vi "Config main.vi"() -> ()   [LabVIEW 2025]
panel:
  in  "Profile Creation":bool
  in  "BATTERY EMULATOR":bool
  in  "CAN CONF":bool
  in  "Configuration":bool
  in  "Home":bool
  in  "Data Log":bool
  in  "Limit Config":bool
  in  "Calibration1":bool
  in  "IO Config":bool
  # "CONFIGURATION"
  # "SETTINGS"
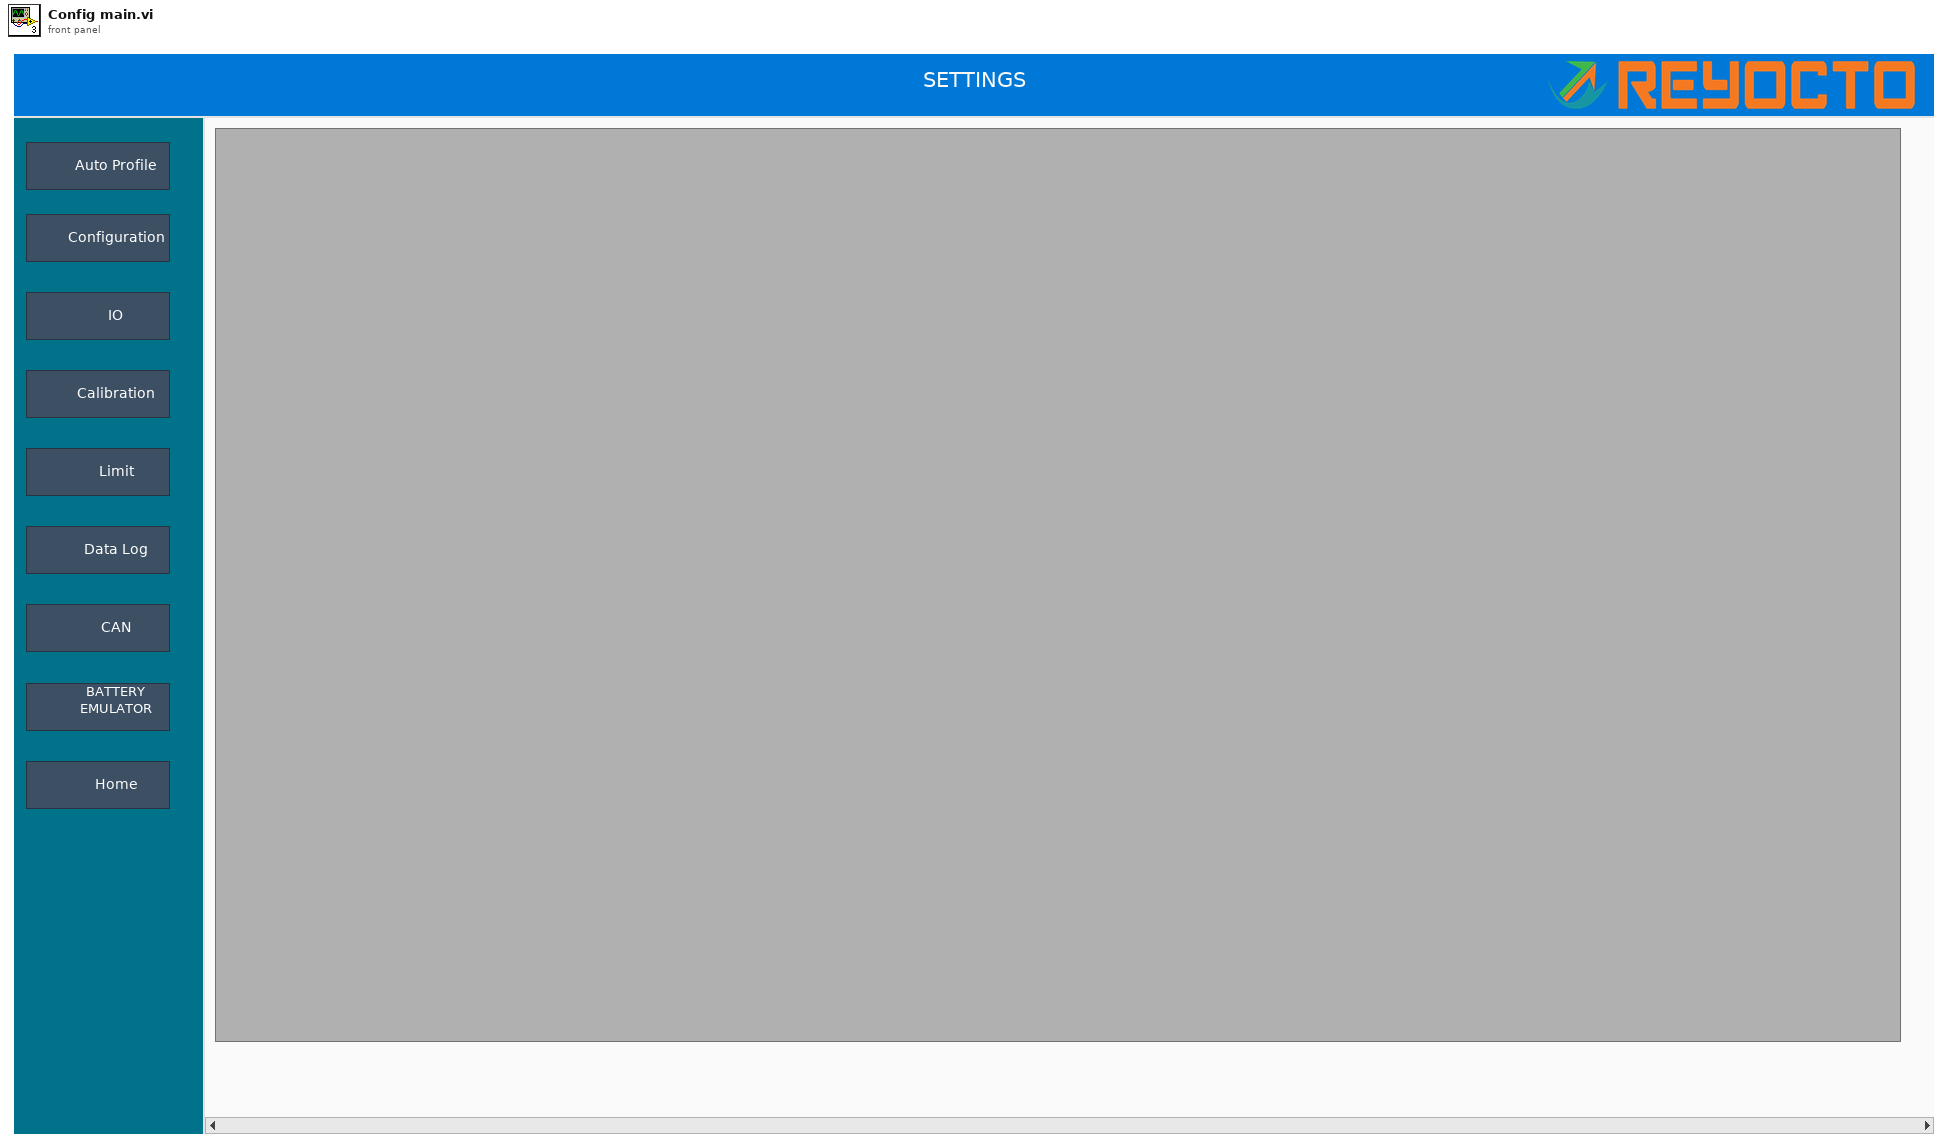
[diagram p1: front panel]
types:
  T1 = enum32{"invalid app kind", "Development System", "Run Time System", "Student Edition", "Embedded LabVIEW", "Evaluation", "Custom"}
  T2 = enum32{"Invalid", "Standard", "Closed", "Hidden", "Minimized", "Maximized"}
  T3 = cluster{"Core":cluster{"Current VI Reference":refnum<vi>, "Close Panel on Exit?":bool}, "Sub Panel":refnum<vi>, "Slected VI":string, "Vi Path":path}
  T4 = cluster{"Current VI Reference":refnum<vi>, "Close Panel on Exit?":bool}
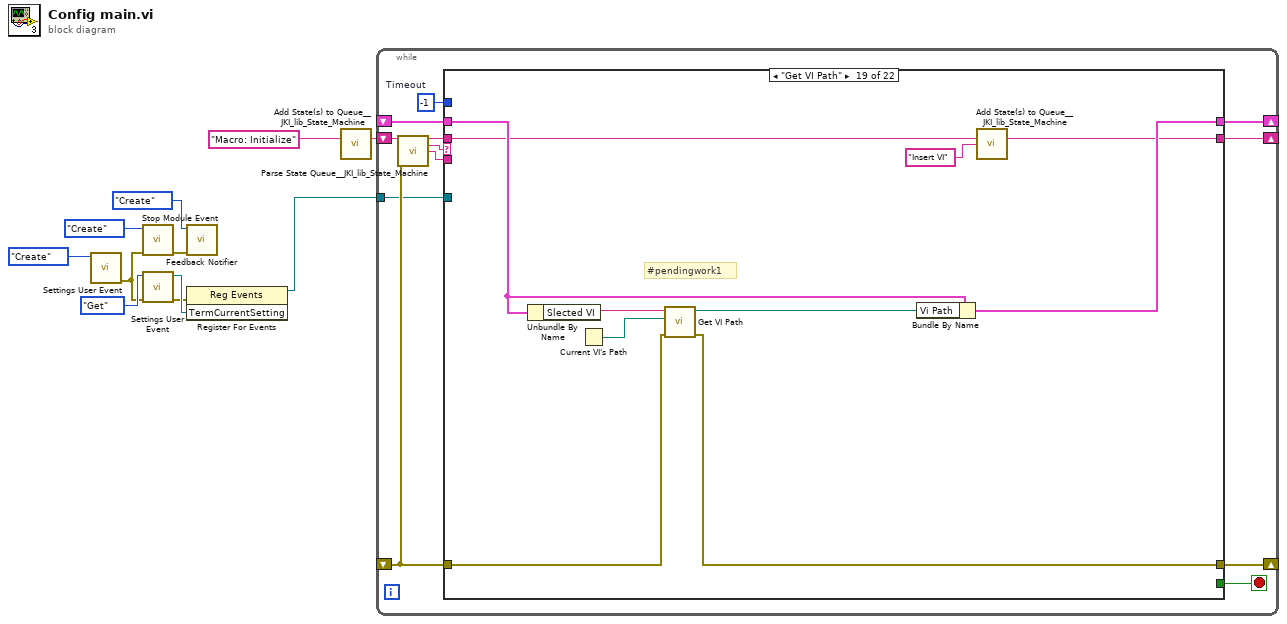
[diagram p0: block diagram]
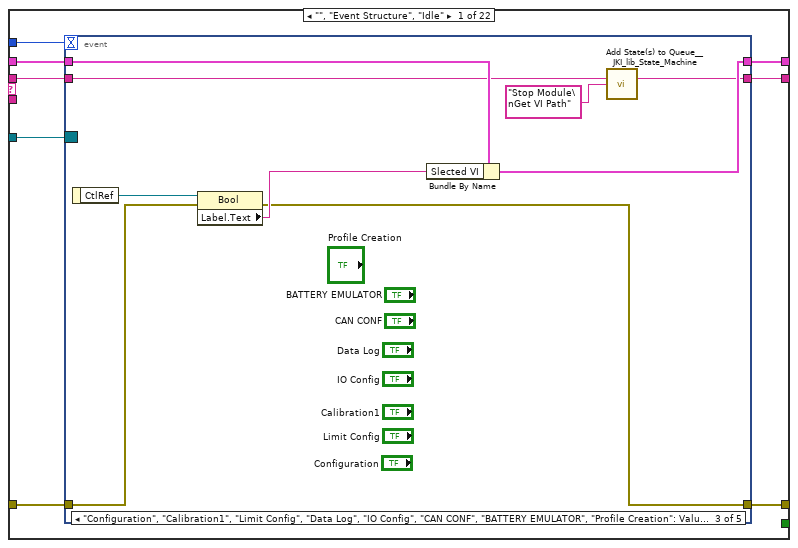
[diagram p2: hidden frame]
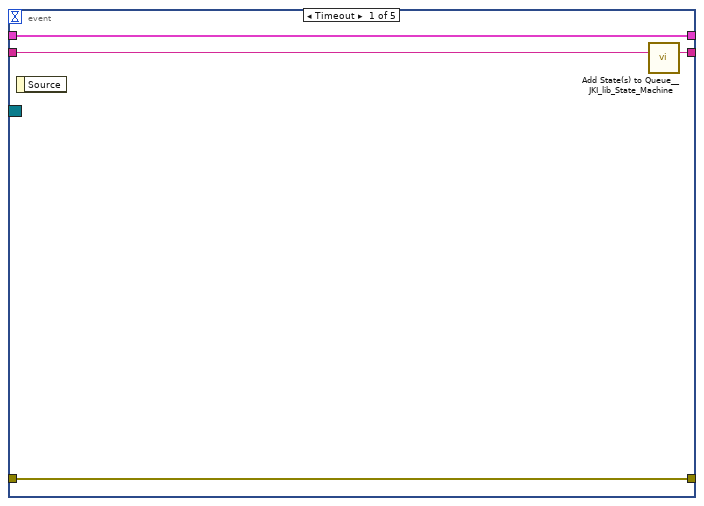
[diagram p3: hidden frame]
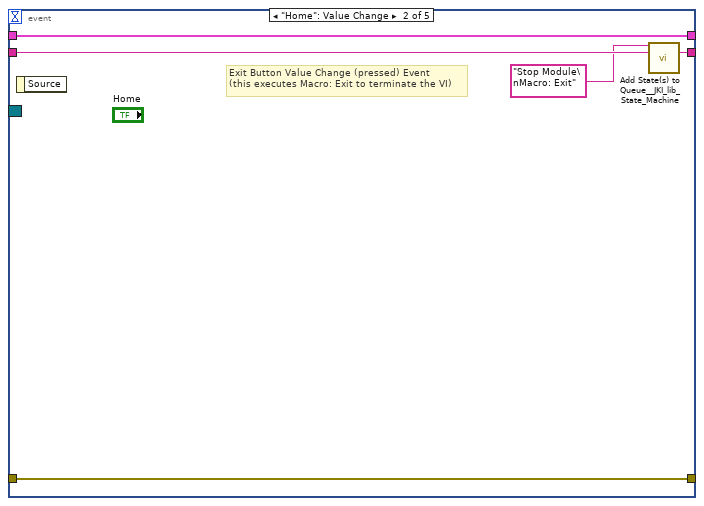
[diagram p4: hidden frame]
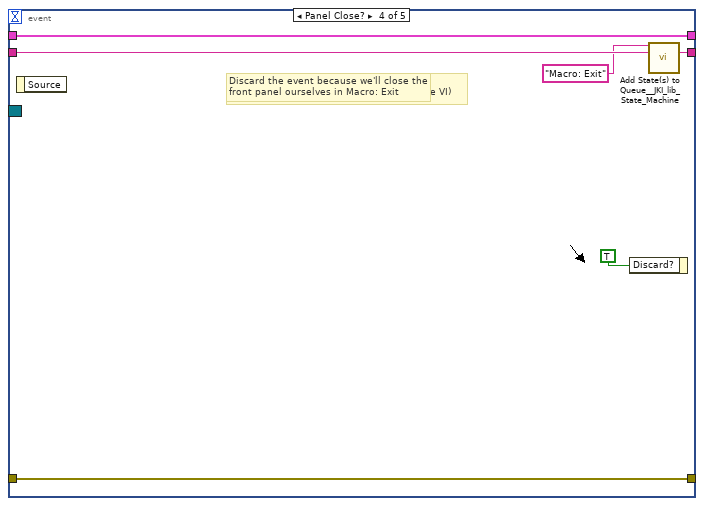
[diagram p5: hidden frame]
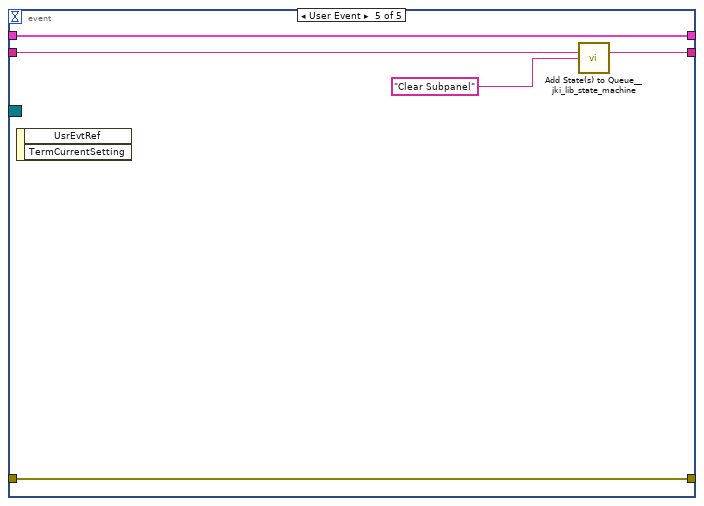
[diagram p6: hidden frame]
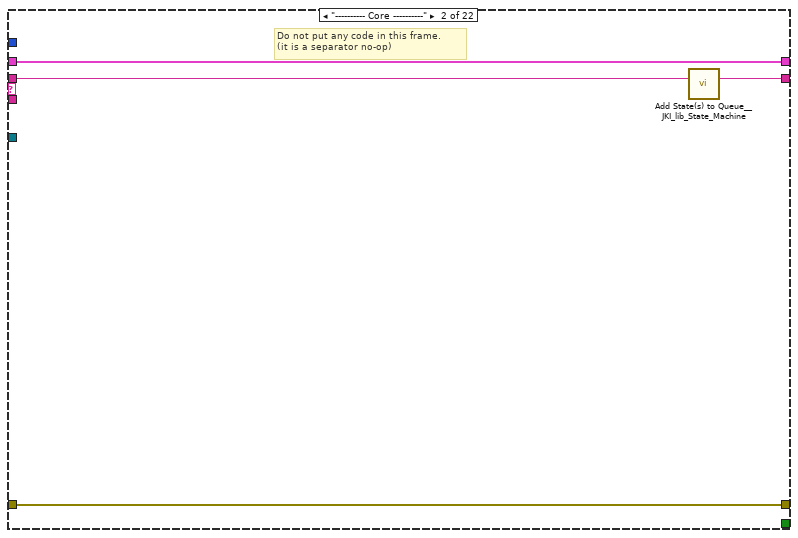
[diagram p7: hidden frame]
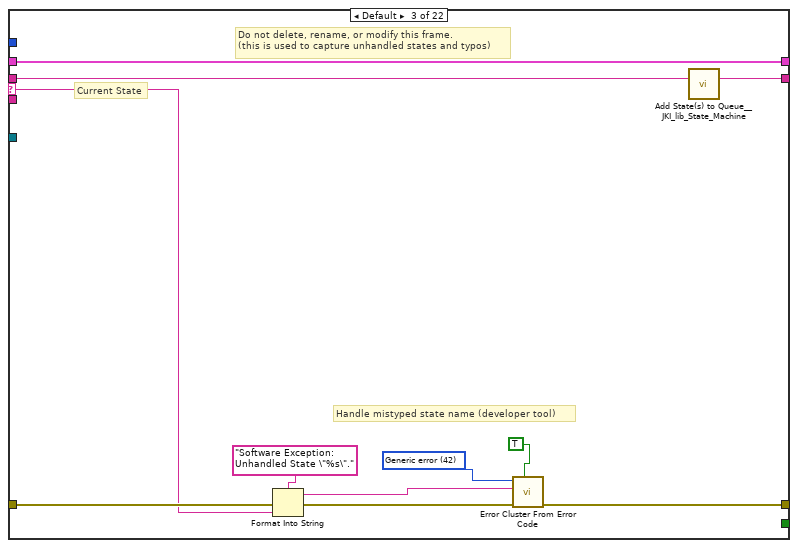
[diagram p8: hidden frame]
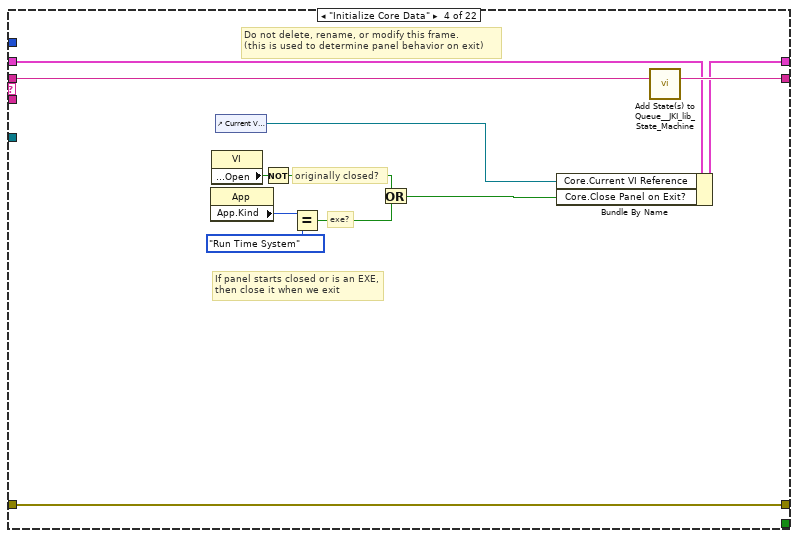
[diagram p9: hidden frame]
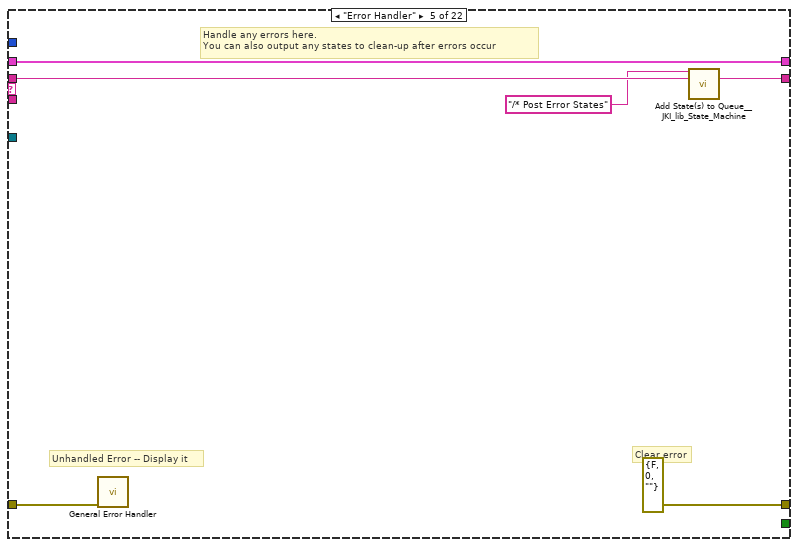
[diagram p10: hidden frame]
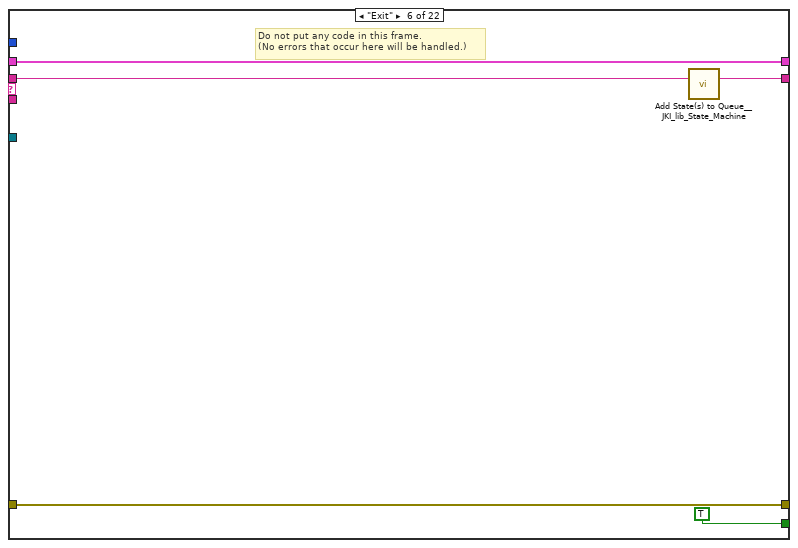
[diagram p11: hidden frame]
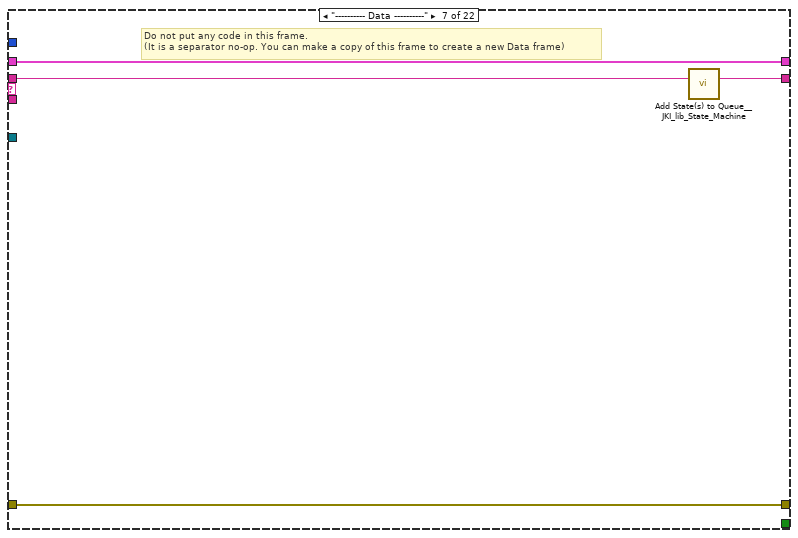
[diagram p12: hidden frame]
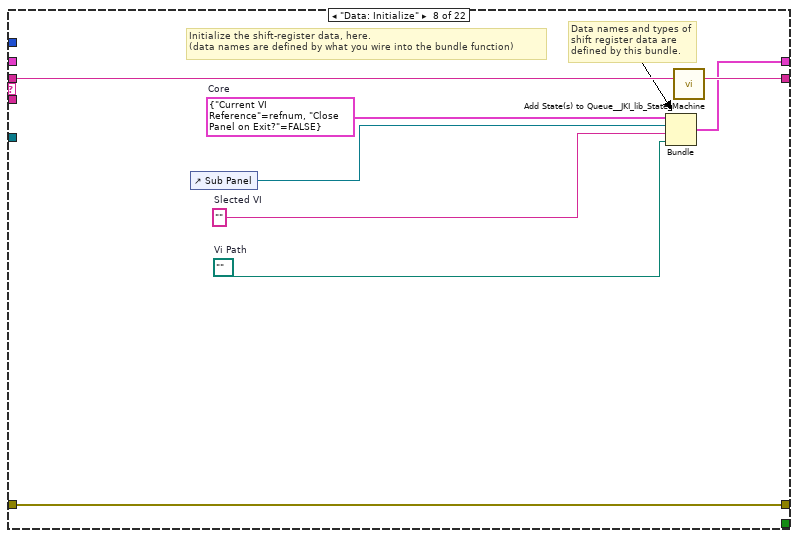
[diagram p13: hidden frame]
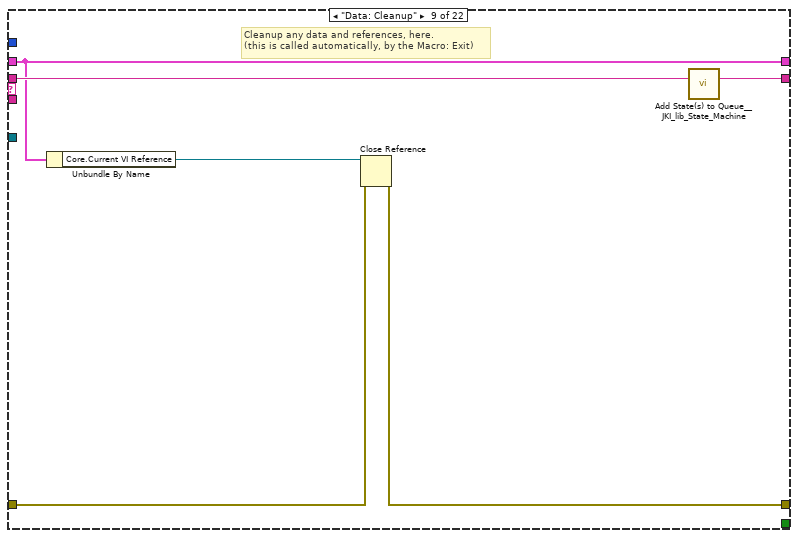
[diagram p14: hidden frame]
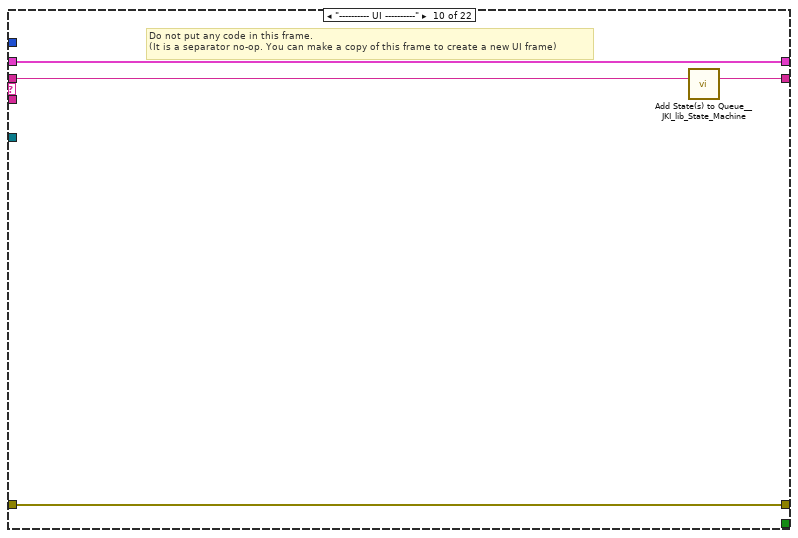
[diagram p15: hidden frame]
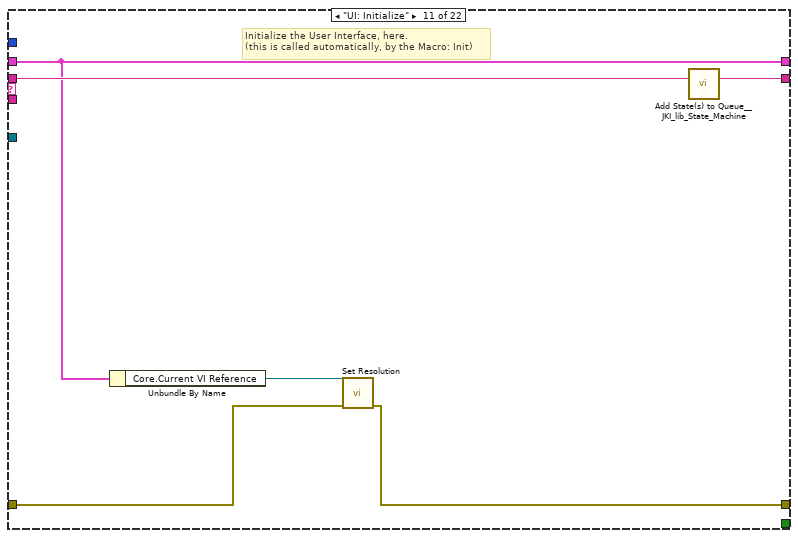
[diagram p16: hidden frame]
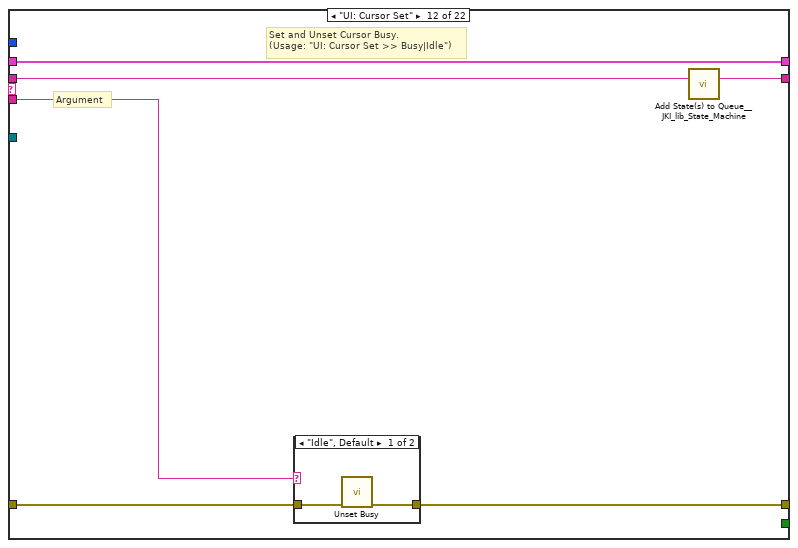
[diagram p17: hidden frame]
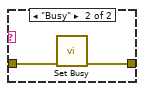
[diagram p18: hidden frame]
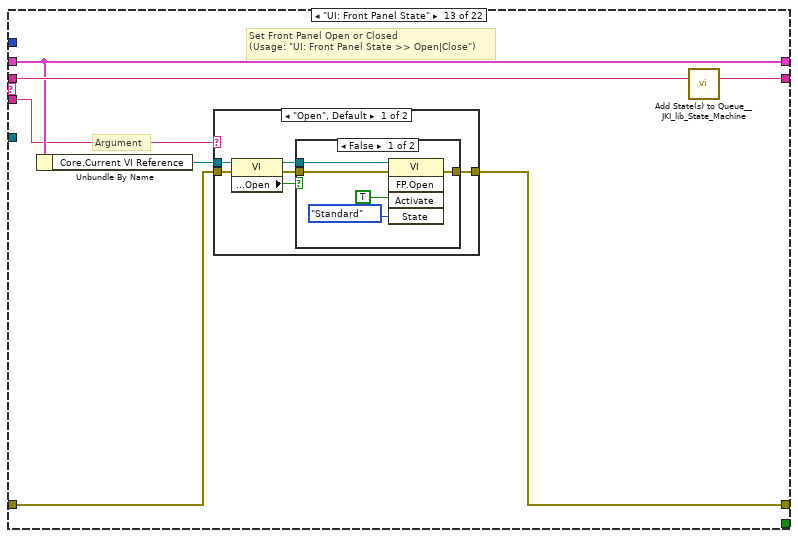
[diagram p19: hidden frame]
diagram:
  n1 = call "Settings User Event.vi"("Action"=enum16{"Create", "Get", "Destroy"}."Create") -> ("error out"=w3:errorcluster)  [unwired: 9 in, 1 out]
  n2 = call "Stop Module Event.vi"("error in (no error)"=w3, "Action"=enum16{"Create", "Get", "Destroy"}."Create") -> ("error out"=w2:errorcluster)  [unwired: 8 in, 1 out]
  n3 = call "Settings User Event.vi"("error in (no error)"=w3, "Action"=enum16{"Create", "Get", "Destroy"}."Get") -> ("error out"=w5:errorcluster, "TermCurrentSetting"=w6:refnum<user-event>)  [unwired: 8 in]
  n4 = call "Feedback Notifier.vi"("error in (no error)"=w2, "Action"=enum16{"Create", "Get", "Destroy"}."Create") -> ()  [unwired: 8 in, 2 out]
  n5 = register-events(error in=w5, w6) -> (reference out=w8:refnum<event-registration>)  [unwired: 1 in, 1 out]
  n6 = call <vilib>:"Add State(s) to Queue__JKI_lib_State_Machine.vi"("State(s) in (\"\")"="Macro: Initialize") -> ("States Out"=w11:string)  [unwired: 14 in]
  n7 = while "JKI - String-Based Queued State Machine (Basic) v1.0" {
    shift-right: [w16] -> _
    shift-left: _ -> [w15]
    shift-right: [w19] -> _
    shift-left: _ -> [w13]
    shift-right: [w18] -> _
    shift-left: w11 -> [w20]
    tunnel: w8 -> [w12]
    stop <- w17 stop-if-true
    w14 = -1  # Timeout
    n8 = call <vilib>:"Parse State Queue__JKI_lib_State_Machine.vi"("State Queue"=w20, "Error In (no error)"=w13) -> ("Remaining States"=w22:string, "Current State"=w23:string, "Arguments"=w21:string)  [unwired: 11 in]
    n9 = case shown="\"Get VI Path\"" w23 {
      selector: w23 -> [_ _ w65 _ _ _ _ _ _ _ _ _ _ _ _ _ _ _ _ _ _ _]
      tunnel: w22 -> [w31 w64 w69 w87 w93 w98 w102 w110 w116 w120 w126 w132 w143 w169 w174 w184 w188 w196 w211 w229 w234 w238]
      tunnel: w21 -> [_ _ _ _ _ _ _ _ _ _ _ w127 w137 _ _ _ _ _ _ _ _ _]
      tunnel: w15 -> [w29 w61 w67 w78 w90 w96 w99 _ w111 w117 w122 w130 w139 w166 w171 w181 w185 w194 w215 w227 w233 w235]
      tunnel: [w28 w62 w71 w84 errorcluster {"status"=FALSE, "code"=0, "source"=""} ("error out") w95 w100 w103 w112 w118 w123 w128 w140 w167 w172 w182 w186 w189 w216 w224 w230 w236] -> w19
      tunnel: w13 -> [w27 w62 w70 w84 w89 w95 w100 w103 w113 w118 w124 w129 w141 w167 w172 w182 w186 w195 w217 w223 w231 w236]
      tunnel: [w30 w63 w68 w86 w92 w97 w101 w109 w115 w119 w125 w131 w142 w168 w173 w183 w187 w196 w210 w228 w234 w237] -> w18
      tunnel: [_ _ _ _ _ TRUE _ _ _ _ _ _ _ _ _ _ _ _ _ _ _ _] -> w17
      tunnel: [w26 w61 w67 w85 w90 w96 w99 w108 w111 w117 w122 w130 w139 w166 w171 w181 w185 w194 w213 w227 w233 w235] -> w16
      tunnel: w14 -> [w25 _ _ _ _ _ _ _ _ _ _ _ _ _ _ _ _ _ _ _ _ _]
      tunnel: w12 -> [w24 _ _ _ _ _ _ _ _ _ _ _ _ _ _ _ _ _ _ _ _ _]
      frame "", "Event Structure", "Idle" {
        n10 = event shown="[2] \"Configuration\", \"Calibration1\", \"Limit Config\", \"Data Log\", \"IO Config\", \"CAN CONF\", \"BATTERY EMULATOR\", \"Profile Creation\": Value Change" {
          selector: w24 -> [_ _ _ _ _]
          dyn-events: _ -> [_ _ _ _ _]
          timeout: w25 -> [_ _ _ _ _]
          tunnel: w31 -> [w35 w40 w44 w55 w57]
          tunnel: [w34 w39 w43 w54 w58] -> w30
          tunnel: w29 -> [w32 w37 w47 w52 w60]
          tunnel: [w33 w38 w41 w53 w59] -> w28
          tunnel: w27 -> [w33 w38 w48 w53 w59]
          tunnel: [w32 w37 w45 w52 w60] -> w26
          event Timeout {
            n11 = event-data() -> ()  [unwired: 1 in, 1 out]
            n12 = call <vilib>:"Add State(s) to Queue__JKI_lib_State_Machine.vi"("State(s) in (\"\")"=w35) -> ("States Out"=w34:string)  [unwired: 14 in]
          }
          event "Home": Value Change {
            # "Exit Button Value Change (pressed) Event\n(this executes Macro: Exit to terminate the VI)"
            n13 = event-data() -> ()  [unwired: 1 in, 1 out]
            n14 = call <vilib>:"Add State(s) to Queue__JKI_lib_State_Machine.vi"("State(s) in Front (\"\")"="Stop Module\nMacro: Exit", "State(s) in (\"\")"=w40) -> ("States Out"=w39:string)  [unwired: 13 in]
          }
          event "Configuration", "Calibration1", "Limit Config", "Data Log", "IO Config", "CAN CONF", "BATTERY EMULATOR", "Profile Creation": Value Change {
            n15 = event-data() -> ("CtlRef"=w49:refnum<vi>)  [unwired: 1 in]
            n16 = property class="Bool"(reference=w49, error in=w48) -> (error out=w41:errorcluster, "Label.Text"=w46:string)  [unwired: 1 out]
            n17 = Bundle By Name(cluster=w47, "Slected VI"=w46) -> (w45:T3)
            n18 = call <vilib>:"Add State(s) to Queue__JKI_lib_State_Machine.vi"("State(s) in (\"\")"=w44, "State(s) at Back (\"\")"="Stop Module\nGet VI Path" ("State(s) at Back (\"\")")) -> ("States Out"=w43:string)  [unwired: 13 in]
          }
          event Panel Close? {
            # "Discard the event because we'll close the front panel ourselves in Macro: Exit"
            # "Close Panel button (pressed) Event\n(this executes Macro: Exit to terminate the VI)"
            n19 = event-data() -> ()  [unwired: 1 in, 1 out]
            n20 = event-data("Discard?"=TRUE) -> ()  [unwired: 1 in, 1 out]
            n21 = call <vilib>:"Add State(s) to Queue__JKI_lib_State_Machine.vi"("State(s) in Front (\"\")"="Macro: Exit", "State(s) in (\"\")"=w55) -> ("States Out"=w54:string)  [unwired: 13 in]
          }
          event User Event {
            n22 = event-data() -> ()  [unwired: 1 in, 2 out]
            n23 = call <vilib>:"Add State(s) to Queue__jki_lib_state_machine.vi"("State(s) in (\"\")"=w57, "State(s) at Back (\"\")"="Clear Subpanel" ("State(s) at Back (\"\")")) -> ("States Out"=w58:string)  [unwired: 13 in]
          }
        }
      }
      frame "---------- Core ----------" {
        # "Do not put any code in this frame.\n(it is a separator no-op)"
        n24 = call <vilib>:"Add State(s) to Queue__JKI_lib_State_Machine.vi"("State(s) in (\"\")"=w64) -> ("States Out"=w63:string)  [unwired: 14 in]
      }
      frame Default {
        w74 = 42 items=["No error", "Argument error", "Memory is full", "Out of zone", "End of file", "File already open", "Generic file I/O error", "File not found", "File permission error", "Disk is full", "Duplicate path", "Too many files open", "System feature not enabled", "Resource file not found", "Cannot add resource", "Resource not found", "Image not found", "Image memory error", "Pen does not exist", "Config type invalid", "Config token not found", "Config parse error", "Config memory error", "Bad external code format", "Bad external code offset", "External code not present", "Null window", "Destroy window error", "Null menu", "Print aborted", "Bad print record", "Print driver error", "Windows error during printing", "Memory error during printing", "Print dialog error", "Generic print error", "Invalid device refnum", "Device not found", "Device parameter error", "Device unit error", "Cannot open device", "Device call aborted", "Generic error", "Cancelled by user", "Object ID too low", "Object ID too high", "Object not in heap", "Unknown heap", "Unknown object (invalid DefProc)", "Unknown object (DefProc not in table)", "Message out of range", "Invalid (null) method", "Unknown message", "Manager call not supported", "Bad address", "Network operation in progress", "Network operation timed out", "Connection is busy", "Network attribute not supported", "Network error", "Address in use", "System out of memory", "Connection aborted", "Connection refused", "Not connected", "Already connected", "Connection closed", "Initialization error (interapplication manager)", "Bad occurrence", "Wait on unbound occurrence handler", "Occurrence queue overflow", "Datalog type conflict", "Unused", "Unrecognized type (interapplication manager)", "Memory corrupt", "Failed to make temporary DLL", "Old CIN version", "Drag socket not found", "Failed to load drop-object", "Failed to register OLE object", "Failed to release OLE object", "Format specifier type mismatch", "Unknown format specifier", "Too few format specifiers", "Too many format specifiers", "Scan failed", "Newer CIN version", "Error converting to variant", "Runtime menu error", "Password tampered", "Variant attribute not found", "Incompatible variant data type", "Event data is not available", "Event Store is not present", "Occurrence is not found", "Event Queue is not created", "Event info is not available", "Refnum passed is NULL", "Error retrieving Class GUID", "Error retrieving CoClass GUID", "Error retrieving TypeLib GUID.", "Bad built application magic bytes.", "Specific driver is different from the specific driver associated with the Logical Name.", "There is no session opened to the class driver.", "Max Error", "MAX - Error with config objects", "MAX - Error loading configuration", "MAX - Group not supported"]
        # "Current State"
        # "Do not delete, rename, or modify this frame.\n(this is used to capture unhandled states and typos)"
        # "Handle mistyped state name (developer tool)"
        n25 = Format Into String(format string="Software Exception: Unhandled State \"%s\"." ("message"), error in=w70, w65) -> (resulting string=w73:string, error out=w72:errorcluster)  [unwired: 1 in]
        n26 = call <vilib>:"Error Cluster From Error Code.vi"("show call chain? (False)"=TRUE, "error in (no error)"=w72, "error message (\"\")"=w73, "error code (0)"=w74) -> ("error out"=w71:errorcluster)  [unwired: 5 in]
        n27 = call <vilib>:"Add State(s) to Queue__JKI_lib_State_Machine.vi"("State(s) in (\"\")"=w69) -> ("States Out"=w68:string)  [unwired: 14 in]
      }
      frame "Initialize Core Data" {
        # "Do not delete, rename, or modify this frame.\n(this is used to determine panel behavior on exit)"
        # "originally closed?"
        # "exe?"
        # "If panel starts closed or is an EXE, then close it when we exit"
        n28 = property class="App"() -> ("App.Kind"=w82:T1)  [unwired: 2 in, 2 out]
        n29 = property class="VI"() -> ("Front Panel.Open"=w83:bool)  [unwired: 2 in, 2 out]
        n30 = control-ref of="Current VI Reference"() -> (w76:refnum<vi>)
        n31 = Not(x=w83) -> (.not. x?=w80:bool)
        n32 = Equal?(x=w82, y=T1."Run Time System" ("Application:Kind")) -> (x = y?=w79:bool)
        n33 = Or(x=w80, y=w79) -> (x .or. y?=w77:bool)
        n34 = Bundle By Name(cluster=w78, "Core.Current VI Reference"=w76, "Core.Close Panel on Exit?"=w77) -> (w85:T3)
        n35 = call <vilib>:"Add State(s) to Queue__JKI_lib_State_Machine.vi"("State(s) in (\"\")"=w87) -> ("States Out"=w86:string)  [unwired: 14 in]
      }
      frame "Error Handler" {
        # "Unhandled Error -- Display it"
        # "Handle any errors here.\nYou can also output any states to clean-up after errors occur"
        # "Clear error"
        n36 = call <vilib>:"General Error Handler.vi"("error in (no error)"=w89) -> ()  [unwired: 10 in, 5 out]
        n37 = call <vilib>:"Add State(s) to Queue__JKI_lib_State_Machine.vi"("State(s) in Front (\"\")"="/* Post Error States", "State(s) in (\"\")"=w93) -> ("States Out"=w92:string)  [unwired: 13 in]
      }
      frame "Exit" {
        # "Do not put any code in this frame.\n(No errors that occur here will be handled.)"
        n38 = call <vilib>:"Add State(s) to Queue__JKI_lib_State_Machine.vi"("State(s) in (\"\")"=w98) -> ("States Out"=w97:string)  [unwired: 14 in]
      }
      frame "---------- Data ----------" {
        # "Do not put any code in this frame.\n(It is a separator no-op. You can make a copy of this frame to create a new Data frame)"
        n39 = call <vilib>:"Add State(s) to Queue__JKI_lib_State_Machine.vi"("State(s) in (\"\")"=w102) -> ("States Out"=w101:string)  [unwired: 14 in]
      }
      frame "Data: Initialize" {
        w105 = path ""  # Vi Path
        w106 = T4 {"Current VI Reference"=refnum, "Close Panel on Exit?"=FALSE}  # Core
        w107 = ""  # Slected VI
        # "Data names and types of shift register data are defined by this bundle."
        # "Initialize the shift-register data, here.\n(data names are defined by what you wire into the bundle function)"
        n40 = control-ref of="Sub Panel"() -> (w104:refnum<vi>)
        n41 = Bundle("Core"=w106, "Sub Panel"=w104, "Slected VI"=w107, "Vi Path"=w105) -> (w108:T3)  [unwired: 1 in]
        n42 = call <vilib>:"Add State(s) to Queue__JKI_lib_State_Machine.vi"("State(s) in (\"\")"=w110) -> ("States Out"=w109:string)  [unwired: 14 in]
      }
      frame "Data: Cleanup" {
        # "Cleanup any data and references, here.\n(this is called automatically, by the Macro: Exit)"
        n43 = Unbundle By Name(w111) -> ("Core.Current VI Reference"=w114:refnum<vi>)
        n44 = Close Reference(reference=w114, error in (no error)=w113) -> (error out=w112:errorcluster)
        n45 = call <vilib>:"Add State(s) to Queue__JKI_lib_State_Machine.vi"("State(s) in (\"\")"=w116) -> ("States Out"=w115:string)  [unwired: 14 in]
      }
      frame "---------- UI ----------" {
        # "Do not put any code in this frame.\n(It is a separator no-op. You can make a copy of this frame to create a new UI frame)"
        n46 = call <vilib>:"Add State(s) to Queue__JKI_lib_State_Machine.vi"("State(s) in (\"\")"=w120) -> ("States Out"=w119:string)  [unwired: 14 in]
      }
      frame "UI: Initialize" {
        # "Initialize the User Interface, here.\n(this is called automatically, by the Macro: Init)"
        n47 = Unbundle By Name(w122) -> ("Core.Current VI Reference"=w121:refnum<vi>)
        n48 = call "Set Resolution.vi"("error in (no error)"=w124, "VI in"=w121) -> ("error out"=w123:errorcluster)  [unwired: 8 in, 1 out]
        n49 = call <vilib>:"Add State(s) to Queue__JKI_lib_State_Machine.vi"("State(s) in (\"\")"=w126) -> ("States Out"=w125:string)  [unwired: 14 in]
      }
      frame "UI: Cursor Set" {
        # "Argument"
        # "Set and Unset Cursor Busy.\n(Usage: \"UI: Cursor Set >> Busy|Idle\")"
        n50 = case shown="\"Idle\", Default" w127 {
          tunnel: w129 -> [w134 w136]
          tunnel: [w133 w135] -> w128
          frame "Idle", Default {
            n51 = call <vilib>:"Unset Busy.vi"("error in (no error)"=w134) -> ("error out"=w133:errorcluster)  [unwired: 10 in]
          }
          frame "Busy" {
            n52 = call <vilib>:"Set Busy.vi"("error in (no error)"=w136) -> ("error out"=w135:errorcluster)  [unwired: 9 in, 1 out]
          }
        }
        n53 = call <vilib>:"Add State(s) to Queue__JKI_lib_State_Machine.vi"("State(s) in (\"\")"=w132) -> ("States Out"=w131:string)  [unwired: 14 in]
      }
      frame "UI: Front Panel State" {
        # "Argument"
        # "Set Front Panel Open or Closed\n(Usage: \"UI: Front Panel State >> Open|Close\")"
        n54 = Unbundle By Name(w139) -> ("Core.Current VI Reference"=w138:refnum<vi>)
        n55 = case shown="\"Open\", Default" w137 {
          tunnel: w141 -> [w147 w160]
          tunnel: [w149 w161] -> w140
          tunnel: w138 -> [w148 w158]
          frame "Open", Default {
            n56 = property class="VI"(reference=w148, error in=w147) -> (reference out=w145:refnum<vi>, error out=w146:errorcluster, "Front Panel.Open"=w144:bool)
            n57 = case shown="False" w144 {
              tunnel: [w152 w155] -> w149
              tunnel: w146 -> [w151 w155]
              tunnel: w145 -> [w150 _]
              frame False {
                n58 = invoke class="VI" method="FP.Open"(reference=w150, error in=w151, "Activate"=TRUE, "State"=T2."Standard") -> (error out=w152:errorcluster)  [unwired: 1 in, 4 out]
              }
              frame True {
              }
            }
          }
          frame "Close" {
            n59 = property class="VI"(reference=w158, error in=w160) -> (reference out=w157:refnum<vi>, error out=w159:errorcluster, "Front Panel.Open"=w156:bool)
            n60 = case shown="True" w156 {
              tunnel: [w162 w165] -> w161
              tunnel: w159 -> [w162 w164]
              tunnel: w157 -> [_ w163]
              frame False {
              }
              frame True {
                n61 = invoke class="VI" method="FP.Close"(reference=w163, error in=w164) -> (error out=w165:errorcluster)  [unwired: 1 in, 2 out]
              }
            }
          }
        }
        n62 = call <vilib>:"Add State(s) to Queue__JKI_lib_State_Machine.vi"("State(s) in (\"\")"=w143) -> ("States Out"=w142:string)  [unwired: 14 in]
      }
      frame "---------- Macro ----------" {
        # "Do not put any code in this frame.\n(It is a separator no-op. You can make a copy of this frame to create a new Macro frame)"
        n63 = call <vilib>:"Add State(s) to Queue__JKI_lib_State_Machine.vi"("State(s) in (\"\")"=w169) -> ("States Out"=w168:string)  [unwired: 14 in]
      }
      frame "Macro: Initialize" {
        # "Initialization Macro\n(This is called once, when the VI starts)"
        n64 = call <vilib>:"Add State(s) to Queue__JKI_lib_State_Machine.vi"("State(s) in Front (\"\")"="Data: Initialize\nInitialize Core Data\nUI: Initialize", "State(s) in (\"\")"=w174) -> ("States Out"=w173:string)  [unwired: 13 in]
      }
      frame "Macro: Exit" {
        # "Exit Macro\n(This is called once, when the VI exits)"
        n65 = Unbundle By Name(w181) -> ("Core.Close Panel on Exit?"=w180:bool)
        n66 = Select(t="UI: Front Panel State >> Close", s=w180, f="") -> (s? t:f=w177:string)
        n67 = call <vilib>:"Add State(s) to Queue__JKI_lib_State_Machine.vi"("State(s) in (\"\")"=w177, "State(s) at Back (\"\")"="Data: Cleanup\nExit") -> ("States Out"=w175:string)  [unwired: 13 in]
        n68 = call <vilib>:"Add State(s) to Queue__JKI_lib_State_Machine.vi"("State(s) in Front (\"\")"=w175, "State(s) in (\"\")"=w184) -> ("States Out"=w183:string)  [unwired: 13 in]
      }
      frame "---------- Main----------" {
        # "Template Separator\n(You can make a copy of, or modify, this frame)"
        n69 = call <vilib>:"Add State(s) to Queue__JKI_lib_State_Machine.vi"("State(s) in (\"\")"=w188) -> ("States Out"=w187:string)  [unwired: 14 in]
      }
      frame "Stop Module" {
        n70 = Unbundle By Name(w194) -> ("Sub Panel"=w193:refnum<vi>)
        n71 = property class="SubPnl"(reference=w193, error in=w195) -> (error out=w190:errorcluster, "InsertedVI"=w192:refnum<vi>)  [unwired: 1 out]
        n72 = Not A Number/Path/Refnum?(number/path/refnum=w192) -> (NaN/Path/Refnum?=w191:bool)
        n73 = case shown="False" w191 {
          tunnel: w190 -> [w204 w208]
          tunnel: [w198 w208] -> w189
          frame False {
            n74 = call "Stop Module Event.vi"("error in (no error)"=w204, "Action"=enum16{"Create", "Get", "Destroy"}."Get") -> ("error out"=w205:errorcluster, "Stop Module"=w206:refnum<user-event>)  [unwired: 8 in]
            n75 = Generate User Event(user event=w206, event data cluster=TRUE, error in=w205) -> (error out=w201:errorcluster)  [unwired: 1 in, 1 out]
            n76 = call "Feedback Notifier.vi"("error in (no error)"=w201, "Action"=enum16{"Create", "Get", "Destroy"}."Get") -> ("error out"=w199:errorcluster, "notifier out"=w200:refnum<notifier>)  [unwired: 8 in]
            n77 = Wait on Notification(notifier=w200, timeout in ms (-1)=1000, error in (no error)=w199) -> (error out=w198:errorcluster)  [unwired: 1 in, 3 out]
          }
          frame True {
          }
        }
      }
      frame "Get VI Path" {
        # "#pendingwork1"
        n78 = Unbundle By Name(w215) -> ("Slected VI"=w218:string)
        n79 = Current VI's Path() -> (path=w212:path)
        n80 = call "Get VI Path.vi"("error in (no error)"=w217, "Base path"=w212, "Selected VI"=w218) -> ("error out"=w216:errorcluster, "VI Path"=w214:path)  [unwired: 7 in]
        n81 = Bundle By Name(cluster=w215, "Vi Path"=w214) -> (w213:T3)
        n82 = call <vilib>:"Add State(s) to Queue__JKI_lib_State_Machine.vi"("State(s) in (\"\")"=w211, "State(s) at Back (\"\")"="Insert VI" ("State(s) at Back (\"\")")) -> ("States Out"=w210:string)  [unwired: 13 in]
      }
      frame "Insert VI" {
        n83 = Unbundle By Name(w227) -> ("Vi Path"=w225:path, "Sub Panel"=w219:refnum<vi>)
        n84 = call "Run VI Dynamically2.vi"("error in (no error)"=w223, "Vi Path"=w225) -> ("error out"=w221:errorcluster, "vi reference"=w220:refnum<vi>)  [unwired: 8 in]
        n85 = invoke class="SubPnl" method="Remove VI"(reference=w219, error in=w221) -> (reference out=w226:refnum<vi>, error out=w222:errorcluster)  [unwired: 1 in, 1 out]
        n86 = invoke class="SubPnl" method="Insert VI"(reference=w226, error in=w222, "VI Ref"=w220) -> (error out=w224:errorcluster)  [unwired: 1 in, 3 out]
        n87 = call <vilib>:"Add State(s) to Queue__JKI_lib_State_Machine.vi"("State(s) in (\"\")"=w229) -> ("States Out"=w228:string)  [unwired: 14 in]
      }
      frame "Clear Subpanel" {
        n88 = Unbundle By Name(w233) -> ("Sub Panel"=w232:refnum<vi>)
        n89 = invoke class="SubPnl" method="Remove VI"(reference=w232, error in=w231) -> (error out=w230:errorcluster)  [unwired: 1 in, 2 out]
      }
      frame "New Category: 2" {
        # "Your code here.\n(You can make a copy of, or modify, this frame)"
        n90 = call <vilib>:"Add State(s) to Queue__JKI_lib_State_Machine.vi"("State(s) in (\"\")"=w238) -> ("States Out"=w237:string)  [unwired: 14 in]
      }
    }
  }
